vi "Decimate 2D Absolute.vi"(6 "Width":i32, 8 "error in (no error)":errorcluster, 9 "Xmin":i32, 10 "Xmax":i32, 11 "Data to Decimate":dbl[][](array[numeric])) -> (0 "error out":errorcluster, 3 "Decimated Data":dbl[][](array[numeric]))   [LabVIEW 2022 SP3, in "Decimation.lvlib"]
doc: "Decimate 2D array to optimize the density of points per pixel to 2 : Min & Max per pixel."
uses:
  Decimation.lvlib
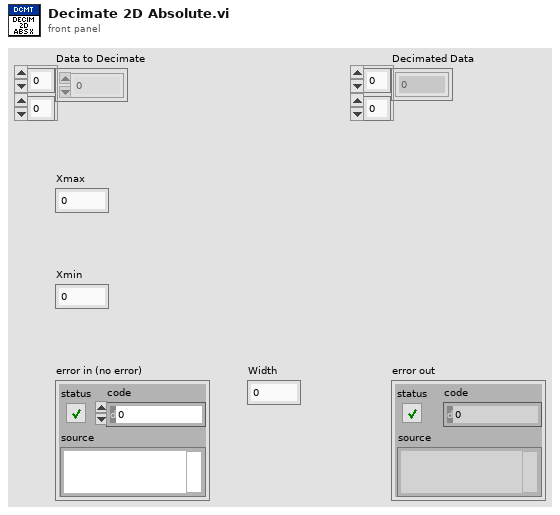
[diagram p1: front panel]
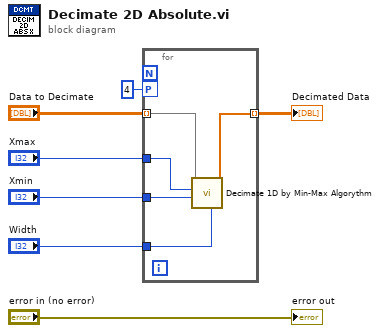
[diagram p0: block diagram]
diagram:
  n1 = for {
    tunnel: "Data to Decimate" -> [w11] mode=indexing
    workers-P: 4 -> [_]
    tunnel: [w12] -> w3 mode=indexing
    tunnel: "Width" -> [w8]
    tunnel: "Xmax" -> [w10]
    tunnel: "Xmin" -> [w9]
    n2 = call "Decimate 1D by Min-Max Algorythm.vi"("Width"=w8, "Min Index"=w9, "Max Index"=w10, "Data To Decimate"=w11) -> ("Decimated Data"=w12:dbl[])  [unwired: 6 in, 1 out]
  }
  "Decimated Data" <- w3
  "error out" <- "error in (no error)"
